vi "Create Cube.vi"() -> (3 "Cube":T1 {"Triangles"."Vertex 3"."UV"."v" min=0 max=1 step=0.1; "Triangles"."Vertex 3"."UV"."u" min=0 max=1 step=0.1; "Triangles"."Vertex 2"."UV"."v" min=0 max=1 step=0.1; "Triangles"."Vertex 2"."UV"."u" min=0 max=1 step=0.1; "Triangles"."Vertex 1"."UV"."v" min=0 max=1 step=0.1; "Triangles"."Vertex 1"."UV"."u" min=0 max=1 step=0.1})   [LabVIEW 2020, in "3D (FPGA).lvlib"]
uses:
  3D (FPGA).lvlib
  Vector 3D.ctl
  Triangle 3D.ctl
  Object.ctl
  Raster/Rectangle Dimensions.ctl
  Raster/Raster (FPGA).lvlib
  Raster/Texture.ctl
  Material.ctl
  Transform.ctl
  Raster/UV.ctl
  Vertex.ctl
  Triangle.ctl
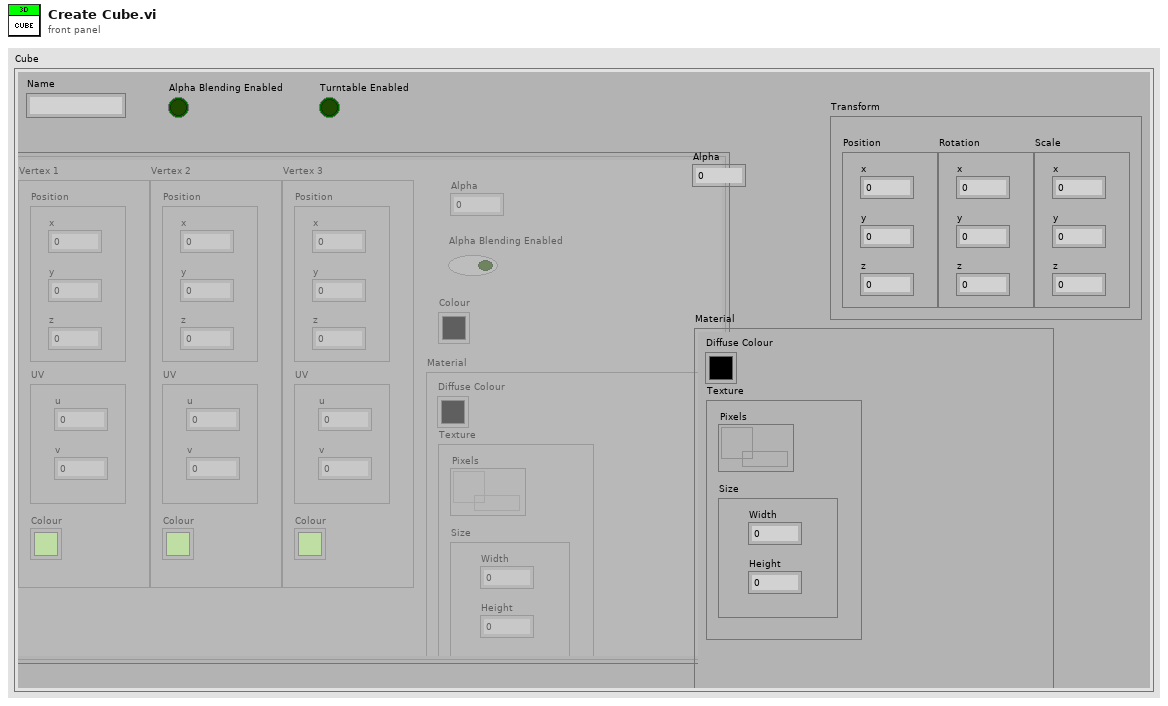
[diagram p1: front panel]
types:
  T1 = typedef "3D (FPGA).lvlib/Object.ctl" = cluster{"Triangles":T2[], "Transform":T9, "Name":string, "Alpha Blending Enabled":bool, "Alpha":dbl, "Turntable Enabled":bool, "Material":T6}
  T2 = typedef "3D (FPGA).lvlib/Triangle.ctl" = cluster{"Vertex 1":T3, "Vertex 2":T3, "Vertex 3":T3, "Alpha":dbl, "Alpha Blending Enabled":bool, "Colour":u32, "Material":T6}
  T3 = typedef "3D (FPGA).lvlib/Vertex.ctl" = cluster{"Position":T4, "UV":T5, "Colour":u32}
  T4 = typedef "3D (FPGA).lvlib/Vector 3D.ctl" = cluster{"x":sgl, "y":sgl, "z":sgl}
  T5 = typedef "Raster (FPGA).lvlib/UV.ctl" = cluster{"u":sgl, "v":sgl}
  T6 = typedef "3D (FPGA).lvlib/Material.ctl" = cluster{"Diffuse Colour":u32, "Texture":T7}
  T7 = typedef "Raster (FPGA).lvlib/Texture.ctl" = cluster{"Pixels":refnum<data-value>, "Size":T8}
  T8 = typedef "Raster (FPGA).lvlib/Rectangle Dimensions.ctl" = cluster{"Width":u32, "Height":u32}
  T9 = typedef "3D (FPGA).lvlib/Transform.ctl" = cluster{"Position":T4, "Rotation":T4, "Scale":T4}
  T10 = typedef "3D (FPGA).lvlib/Triangle 3D.ctl" = cluster{"Point 1":T4, "Point 2":T4, "Point 3":T4}
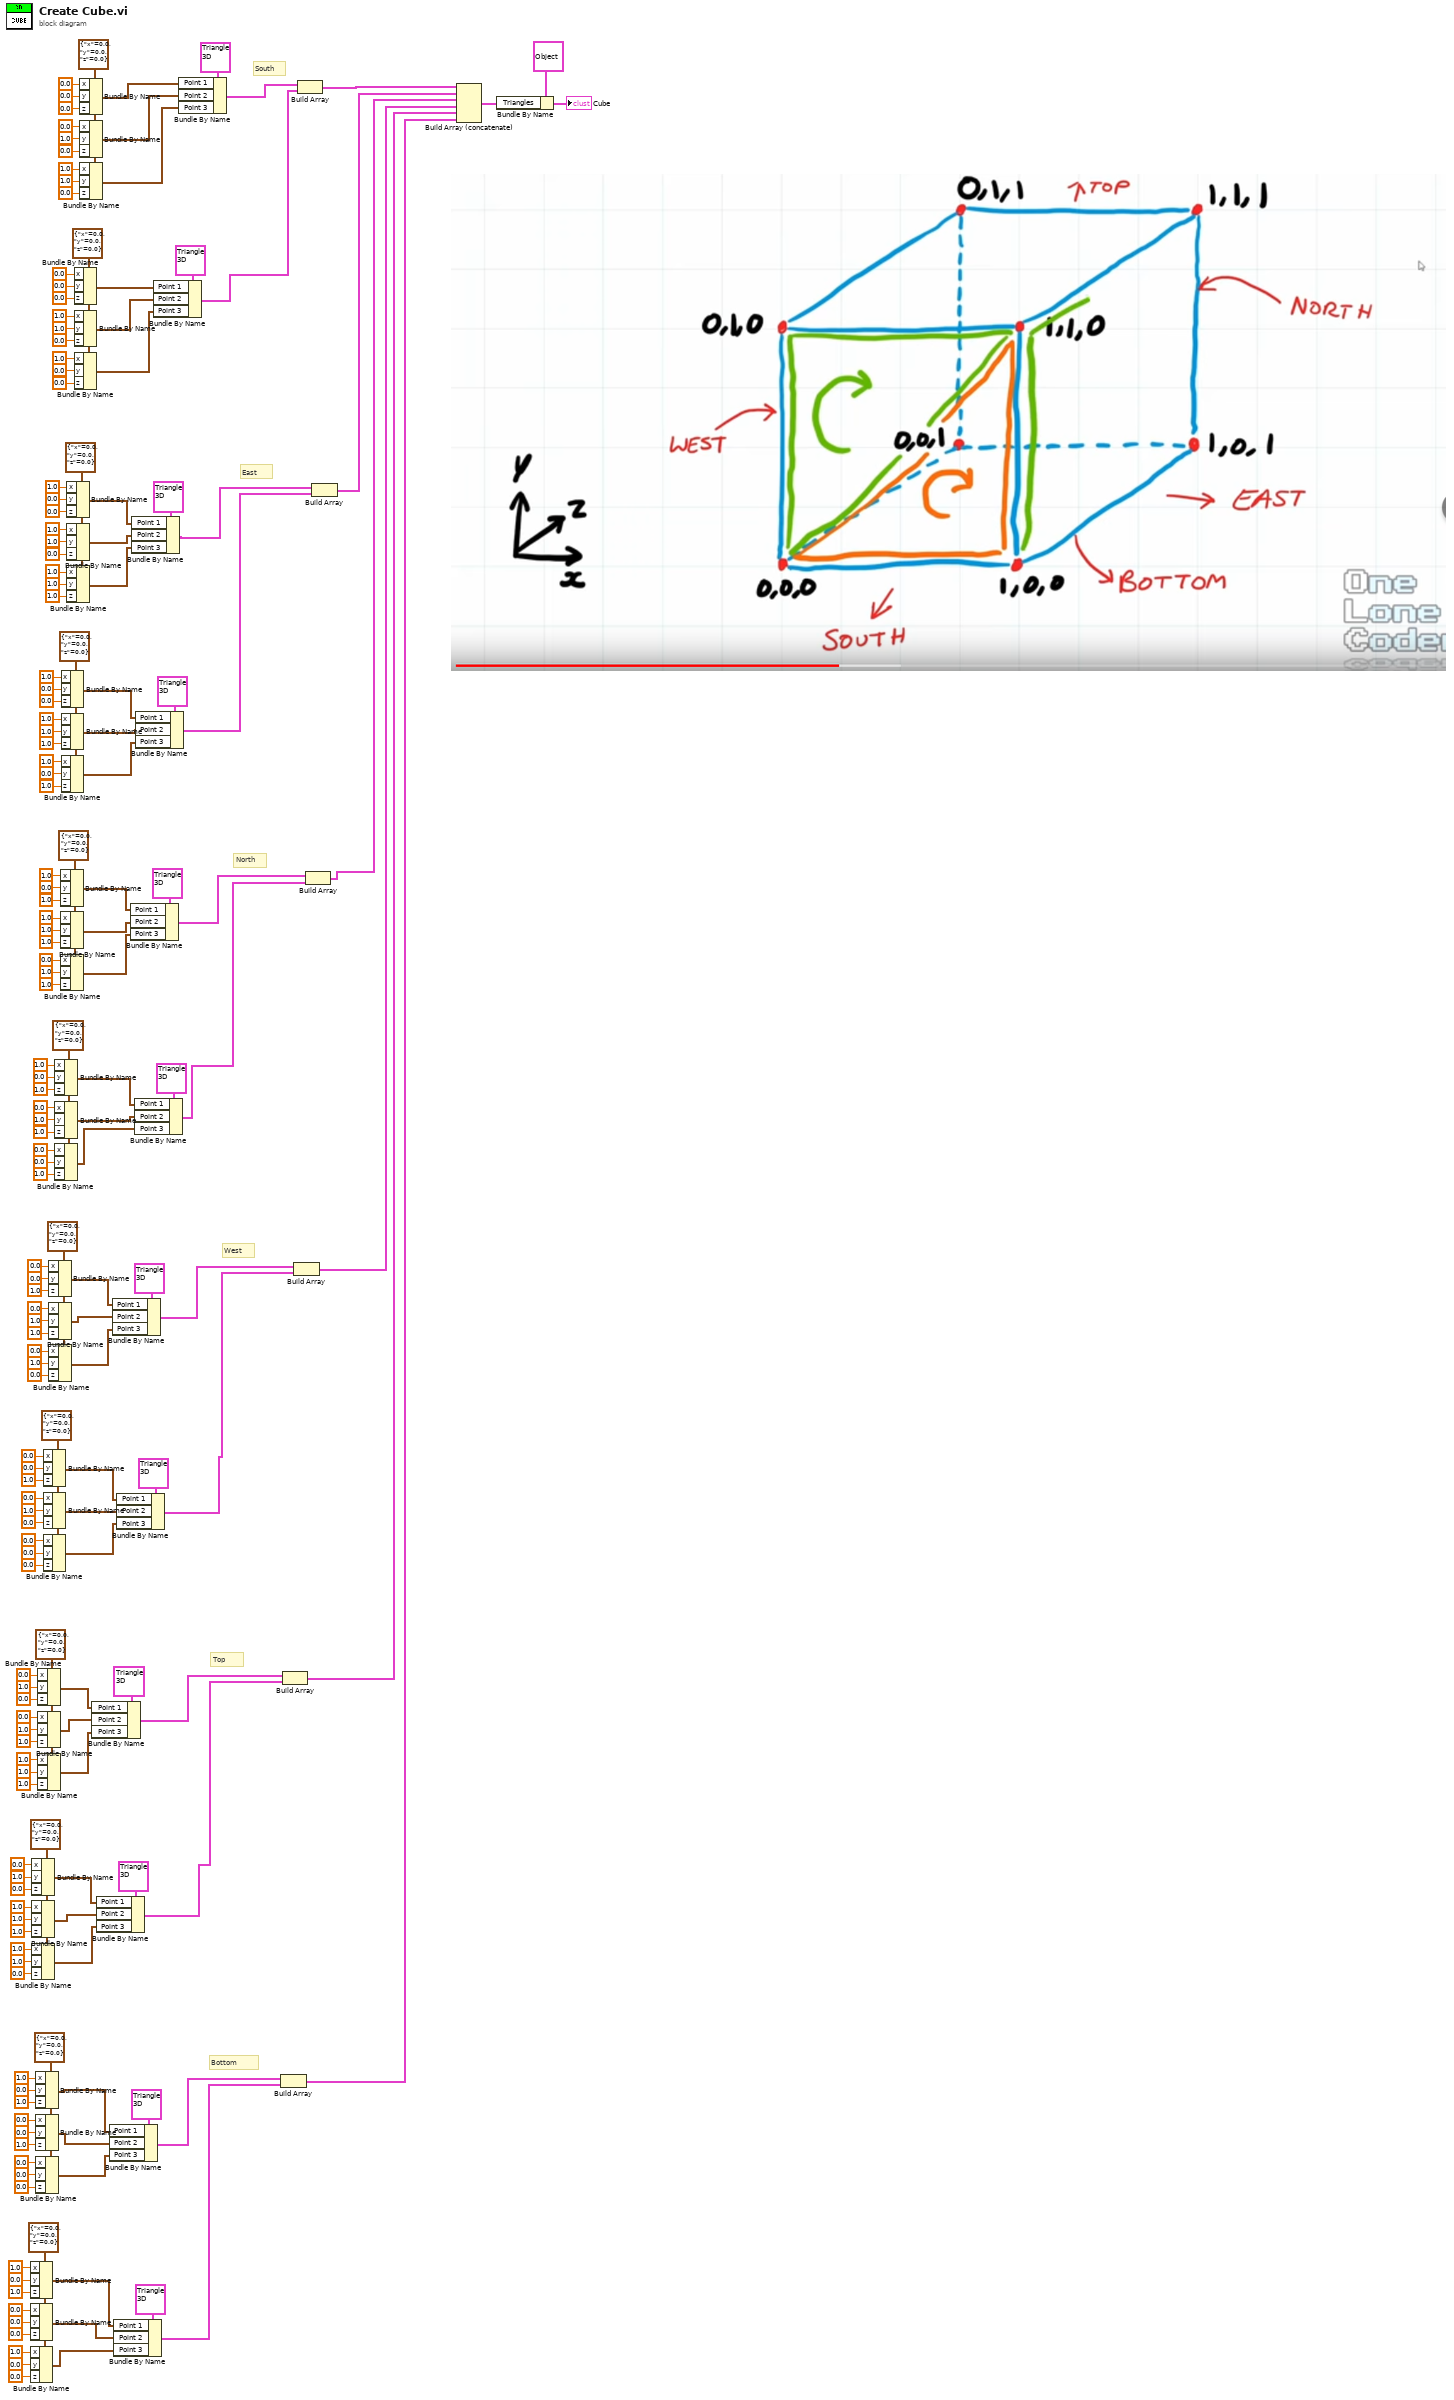
[diagram p0: block diagram]
diagram:
  w76 = T4 {"x"=0.0, "y"=0.0, "z"=0.0} ("Vector 3D")
  w75 = T4 {"x"=0.0, "y"=0.0, "z"=0.0} ("Vector 3D")
  w95 = T4 {"x"=0.0, "y"=0.0, "z"=0.0} ("Vector 3D")
  w96 = T4 {"x"=0.0, "y"=0.0, "z"=0.0} ("Vector 3D")
  w116 = T4 {"x"=0.0, "y"=0.0, "z"=0.0} ("Vector 3D")
  w115 = T4 {"x"=0.0, "y"=0.0, "z"=0.0} ("Vector 3D")
  w135 = T4 {"x"=0.0, "y"=0.0, "z"=0.0} ("Vector 3D")
  w136 = T4 {"x"=0.0, "y"=0.0, "z"=0.0} ("Vector 3D")
  w156 = T4 {"x"=0.0, "y"=0.0, "z"=0.0} ("Vector 3D")
  w155 = T4 {"x"=0.0, "y"=0.0, "z"=0.0} ("Vector 3D")
  w175 = T4 {"x"=0.0, "y"=0.0, "z"=0.0} ("Vector 3D")
  w176 = T4 {"x"=0.0, "y"=0.0, "z"=0.0} ("Vector 3D")
  # "Bottom"
  # "Top"
  # "West"
  # "North"
  # "East"
  # "South"
  n1 = Bundle By Name(cluster=w76, "x"=sgl 1.0, "y"=sgl 0.0, "z"=sgl 1.0) -> (w5:T4)
  n2 = Bundle By Name(cluster=w76, "x"=sgl 0.0, "y"=sgl 0.0, "z"=sgl 0.0) -> (w4:T4)
  n3 = Bundle By Name(cluster=w76, "x"=sgl 1.0, "y"=sgl 0.0, "z"=sgl 0.0) -> (w3:T4)
  n4 = Bundle By Name(cluster=w95, "x"=sgl 0.0, "y"=sgl 1.0, "z"=sgl 0.0) -> (w15:T4)
  n5 = Bundle By Name(cluster=w95, "x"=sgl 1.0, "y"=sgl 1.0, "z"=sgl 1.0) -> (w14:T4)
  n6 = Bundle By Name(cluster=w95, "x"=sgl 1.0, "y"=sgl 1.0, "z"=sgl 0.0) -> (w13:T4)
  n7 = Bundle By Name(cluster=w75, "x"=sgl 1.0, "y"=sgl 0.0, "z"=sgl 1.0) -> (w8:T4)
  n8 = Bundle By Name(cluster=w75, "x"=sgl 0.0, "y"=sgl 0.0, "z"=sgl 1.0) -> (w7:T4)
  n9 = Bundle By Name(cluster=w75, "x"=sgl 0.0, "y"=sgl 0.0, "z"=sgl 0.0) -> (w6:T4)
  n10 = Bundle By Name(cluster=w96, "x"=sgl 0.0, "y"=sgl 1.0, "z"=sgl 0.0) -> (w18:T4)
  n11 = Bundle By Name(cluster=w96, "x"=sgl 0.0, "y"=sgl 1.0, "z"=sgl 1.0) -> (w17:T4)
  n12 = Bundle By Name(cluster=w96, "x"=sgl 1.0, "y"=sgl 1.0, "z"=sgl 1.0) -> (w16:T4)
  n13 = Bundle By Name(cluster=w116, "x"=sgl 0.0, "y"=sgl 0.0, "z"=sgl 1.0) -> (w24:T4)
  n14 = Bundle By Name(cluster=w116, "x"=sgl 0.0, "y"=sgl 1.0, "z"=sgl 0.0) -> (w23:T4)
  n15 = Bundle By Name(cluster=w116, "x"=sgl 0.0, "y"=sgl 0.0, "z"=sgl 0.0) -> (w22:T4)
  n16 = Bundle By Name(cluster=w115, "x"=sgl 0.0, "y"=sgl 0.0, "z"=sgl 1.0) -> (w28:T4)
  n17 = Bundle By Name(cluster=w115, "x"=sgl 0.0, "y"=sgl 1.0, "z"=sgl 1.0) -> (w27:T4)
  n18 = Bundle By Name(cluster=w115, "x"=sgl 0.0, "y"=sgl 1.0, "z"=sgl 0.0) -> (w26:T4)
  n19 = Bundle By Name(cluster=w135, "x"=sgl 1.0, "y"=sgl 0.0, "z"=sgl 1.0) -> (w35:T4)
  n20 = Bundle By Name(cluster=w135, "x"=sgl 0.0, "y"=sgl 1.0, "z"=sgl 1.0) -> (w34:T4)
  n21 = Bundle By Name(cluster=w135, "x"=sgl 0.0, "y"=sgl 0.0, "z"=sgl 1.0) -> (w33:T4)
  n22 = Bundle By Name(cluster=w136, "x"=sgl 1.0, "y"=sgl 0.0, "z"=sgl 1.0) -> (w38:T4)
  n23 = Bundle By Name(cluster=w136, "x"=sgl 1.0, "y"=sgl 1.0, "z"=sgl 1.0) -> (w37:T4)
  n24 = Bundle By Name(cluster=w136, "x"=sgl 0.0, "y"=sgl 1.0, "z"=sgl 1.0) -> (w36:T4)
  n25 = Bundle By Name(cluster=w156, "x"=sgl 1.0, "y"=sgl 0.0, "z"=sgl 0.0) -> (w44:T4)
  n26 = Bundle By Name(cluster=w156, "x"=sgl 1.0, "y"=sgl 1.0, "z"=sgl 1.0) -> (w43:T4)
  n27 = Bundle By Name(cluster=w156, "x"=sgl 1.0, "y"=sgl 0.0, "z"=sgl 1.0) -> (w42:T4)
  n28 = Bundle By Name(cluster=w155, "x"=sgl 1.0, "y"=sgl 0.0, "z"=sgl 0.0) -> (w49:T4)
  n29 = Bundle By Name(cluster=w155, "x"=sgl 1.0, "y"=sgl 1.0, "z"=sgl 0.0) -> (w48:T4)
  n30 = Bundle By Name(cluster=w155, "x"=sgl 1.0, "y"=sgl 1.0, "z"=sgl 1.0) -> (w47:T4)
  n31 = Bundle By Name(cluster=w175, "x"=sgl 0.0, "y"=sgl 0.0, "z"=sgl 0.0) -> (w54:T4)
  n32 = Bundle By Name(cluster=w175, "x"=sgl 1.0, "y"=sgl 1.0, "z"=sgl 0.0) -> (w53:T4)
  n33 = Bundle By Name(cluster=w175, "x"=sgl 1.0, "y"=sgl 0.0, "z"=sgl 0.0) -> (w52:T4)
  n34 = Bundle By Name(cluster=w176, "x"=sgl 0.0, "y"=sgl 0.0, "z"=sgl 0.0) -> (w58:T4)
  n35 = Bundle By Name(cluster=w176, "x"=sgl 0.0, "y"=sgl 1.0, "z"=sgl 0.0) -> (w57:T4)
  n36 = Bundle By Name(cluster=w176, "x"=sgl 1.0, "y"=sgl 1.0, "z"=sgl 0.0) -> (w56:T4)
  n37 = Bundle By Name(cluster=T10 {"Point 1"={"x"=0.0, "y"=0.0, "z"=0.0}, "Point 2"={"x"=0.0, "y"=0.0, "z"=0.0}, "Point 3"={"x"=0.0, "y"=0.0, "z"=0.0}} ("Triangle"), "Point 1"=w18, "Point 2"=w17, "Point 3"=w16) -> (w12:T10)
  n38 = Bundle By Name(cluster=T10 {"Point 1"={"x"=0.0, "y"=0.0, "z"=0.0}, "Point 2"={"x"=0.0, "y"=0.0, "z"=0.0}, "Point 3"={"x"=0.0, "y"=0.0, "z"=0.0}} ("Triangle"), "Point 1"=w15, "Point 2"=w14, "Point 3"=w13) -> (w11:T10)
  n39 = Bundle By Name(cluster=T10 {"Point 1"={"x"=0.0, "y"=0.0, "z"=0.0}, "Point 2"={"x"=0.0, "y"=0.0, "z"=0.0}, "Point 3"={"x"=0.0, "y"=0.0, "z"=0.0}} ("Triangle"), "Point 1"=w8, "Point 2"=w7, "Point 3"=w6) -> (w2:T10)
  n40 = Bundle By Name(cluster=T10 {"Point 1"={"x"=0.0, "y"=0.0, "z"=0.0}, "Point 2"={"x"=0.0, "y"=0.0, "z"=0.0}, "Point 3"={"x"=0.0, "y"=0.0, "z"=0.0}} ("Triangle"), "Point 1"=w28, "Point 2"=w27, "Point 3"=w26) -> (w25:T10)
  n41 = Bundle By Name(cluster=T10 {"Point 1"={"x"=0.0, "y"=0.0, "z"=0.0}, "Point 2"={"x"=0.0, "y"=0.0, "z"=0.0}, "Point 3"={"x"=0.0, "y"=0.0, "z"=0.0}} ("Triangle"), "Point 1"=w5, "Point 2"=w4, "Point 3"=w3) -> (w1:T10)
  n42 = Bundle By Name(cluster=T10 {"Point 1"={"x"=0.0, "y"=0.0, "z"=0.0}, "Point 2"={"x"=0.0, "y"=0.0, "z"=0.0}, "Point 3"={"x"=0.0, "y"=0.0, "z"=0.0}} ("Triangle"), "Point 1"=w24, "Point 2"=w23, "Point 3"=w22) -> (w21:T10)
  n43 = Bundle By Name(cluster=T10 {"Point 1"={"x"=0.0, "y"=0.0, "z"=0.0}, "Point 2"={"x"=0.0, "y"=0.0, "z"=0.0}, "Point 3"={"x"=0.0, "y"=0.0, "z"=0.0}} ("Triangle"), "Point 1"=w38, "Point 2"=w37, "Point 3"=w36) -> (w32:T10)
  n44 = Bundle By Name(cluster=T10 {"Point 1"={"x"=0.0, "y"=0.0, "z"=0.0}, "Point 2"={"x"=0.0, "y"=0.0, "z"=0.0}, "Point 3"={"x"=0.0, "y"=0.0, "z"=0.0}} ("Triangle"), "Point 1"=w49, "Point 2"=w48, "Point 3"=w47) -> (w46:T10)
  n45 = Bundle By Name(cluster=T10 {"Point 1"={"x"=0.0, "y"=0.0, "z"=0.0}, "Point 2"={"x"=0.0, "y"=0.0, "z"=0.0}, "Point 3"={"x"=0.0, "y"=0.0, "z"=0.0}} ("Triangle"), "Point 1"=w35, "Point 2"=w34, "Point 3"=w33) -> (w31:T10)
  n46 = Bundle By Name(cluster=T10 {"Point 1"={"x"=0.0, "y"=0.0, "z"=0.0}, "Point 2"={"x"=0.0, "y"=0.0, "z"=0.0}, "Point 3"={"x"=0.0, "y"=0.0, "z"=0.0}} ("Triangle"), "Point 1"=w44, "Point 2"=w43, "Point 3"=w42) -> (w41:T10)
  n47 = Bundle By Name(cluster=T10 {"Point 1"={"x"=0.0, "y"=0.0, "z"=0.0}, "Point 2"={"x"=0.0, "y"=0.0, "z"=0.0}, "Point 3"={"x"=0.0, "y"=0.0, "z"=0.0}} ("Triangle"), "Point 1"=w54, "Point 2"=w53, "Point 3"=w52) -> (w51:T10)
  n48 = Bundle By Name(cluster=T10 {"Point 1"={"x"=0.0, "y"=0.0, "z"=0.0}, "Point 2"={"x"=0.0, "y"=0.0, "z"=0.0}, "Point 3"={"x"=0.0, "y"=0.0, "z"=0.0}} ("Triangle"), "Point 1"=w58, "Point 2"=w57, "Point 3"=w56) -> (w187:T10)
  n49 = Build Array(w2, w1) -> (w61:T10[])
  n50 = Build Array(w12, w11) -> (w62:T10[])
  n51 = Build Array(w25, w21) -> (w63:T10[])
  n52 = Build Array(w187, w51) -> (w60:T10[])
  n53 = Build Array(w32, w31) -> (w64:T10[])
  n54 = Build Array(w46, w41) -> (w65:T10[])
  n55 = Build Array (concatenate)(w60, w65, w64, w63, w62, w61) -> (w59:T10[])
  n56 = Bundle By Name(cluster=T1 {"Triangles"=[], "Transform"={"Position"={"x"=0.0, "y"=0.0, "z"=0.0}, "Rotation"={"x"=0.0, "y"=0.0, "z"=0.0}, "Scale"={"x"=0.0, "y"=0.0, "z"=0.0}}, "Name"="", "Alpha Blending Enabled"=FALSE, "Alpha"=0.0, "Turntable Enabled"=FALSE, "Material"={"Diffuse Colour"=0, "Texture"={"Pixels"=refnum, "Size"={"Width"=0, "Height"=0}}}} ("Mesh"), "Triangles"=w59) -> (→"Cube":T1)
